vi "FPGA set up.vi"(6 "mirror cycles per frame":i16=256, 7 "enable external trigger":bool, 8 "lasersync":bool, 9 "bitfile name":T1, 10 "Start Delay (Ticks)":i16=1 min=1, 11 "resource name":T3) -> (0 "pixels per frame":i32, 3 "FPGA VI Reference Out":T2, 4 "Actual Depth 3":u32)   [LabVIEW 2012]
doc: "SciScan 1.2 160622"
uses:
  <vilib>/userdefined/High Color/nirio_resource_hc.ctl
  Custom Controls/FPGA reference typedef for 120MHz code.ctl
  Custom Controls/biotfile select.ctl
  <vilib>/FPGAPlugInAG/PXIe-7962R/niLvFpga_Open_PXIe-7962R.vi
  <vilib>/rvi/interface/common/dynamic/niFpgaDynamicAddResources.vi
  <vilib>/FPGAPlugInAG/PXIe-7961R/niLvFpga_Open_PXIe-7961R.vi
  <vilib>/FPGAPlugInAG/Dynamic/niLvFpga_Abort_Dynamic.vi
  <vilib>/Utility/error.llb/Error Cluster From Error Code.vi
  <vilib>/rvi/errors/niLvFpgaAdjustHostInterfaceError.vi
  <vilib>/FPGAPlugInAG/Dynamic/niLvFpga_Run_Dynamic.vi
  <vilib>/rvi/interface/nirviOpenFPGA/nirviOpenFPGA.xnode
  fpga bitfiles/7962with5751_512px_40Mhz.lvbitx
  fpga bitfiles/7962with5751_12kHz_512px_50MHz_4ch.lvbitx
  fpga bitfiles/7962with5751_512px_50Mhz.lvbitx
  fpga bitfiles/7961with5734_1024px_120Mhz or ext lasersync.lvbitx
  fpga bitfiles/7962with5734_1024px_120Mhz or ext lasersync.lvbitx
  fpga bitfiles/7962with5751_12kHz_1024px_2ch_50MHz.lvbitx
  fpga bitfiles/7962with5734_512px_120Mhz or ext lasersync.lvbitx
  fpga bitfiles/7961with5734_512px_120Mhz or ext lasersync.lvbitx
  fpga bitfiles/7962with5751_1536px_2ch_40Mhz.lvbitx
  fpga bitfiles/7962with5751_1536px_2ch_50Mhz.lvbitx
  <vilib>/rvi/interface/nirviMethod/nirviMethod.xnode
  <vilib>/rvi/interface/nirviReadWriteControl/nirviReadWriteControl.xnode
  <vilib>/rvi/errors/niLvFpgaMergeErrorWithErrorCode.vi
  <vilib>/FPGAPlugInAG/Dynamic/niLvFpga_ConfigureFifo_Dynamic.vi
  NiFpgaLv.dll
  <vilib>/rvi/interface/Simulation/niFpgaSimulationCallBeginRW.vi
panel:
  out "IO Module\\User Command Status":u8
  out "Array":bool[](array[boolean])
  in  "Requested Depth":u32=100000000
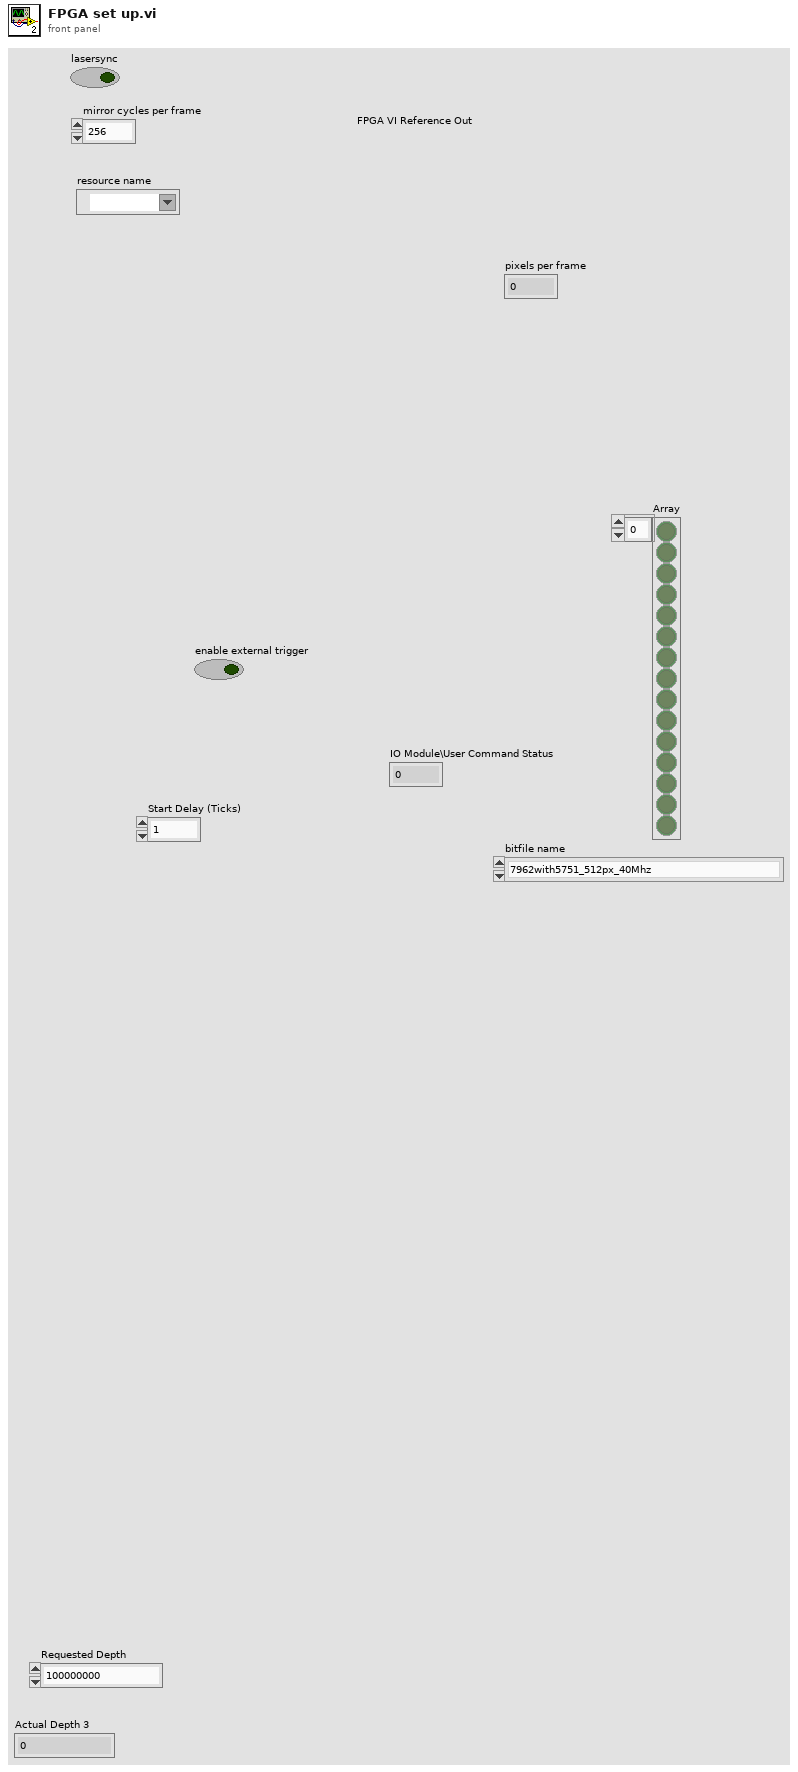
[diagram p1: front panel]
types:
  T1 = typedef "biotfile select.ctl" = enum16{"7962with5751_512px_40Mhz", "7962with5751_512px_50Mhz", "7961with5734_1024px_120Mhz or ext lasersync", "7962with5734_1024px_120Mhz or ext lasersync", "7962with5734_512px_120Mhz or ext lasersync", "7961with5734_512px_120Mhz or ext lasersync", "7962with5751_12kHz_512px_50MHz_4ch", "7962with5751_1536px_2ch_40Mhz", "7962with5751_1536px_2ch_50Mhz", "7962with5751_12kHz_1024px_2ch_50MHz"}
  T2 = typedef "FPGA reference typedef for 120MHz code.ctl" = refnum<k20>
  T3 = typedef "nirio_resource_hc.ctl" = tag
  T4 = cluster{"IO Module\\User Command":u8, "IO Module\\User Data 0":u8, "IO Module\\User Data 1":u8}
  T5 = cluster{"IO Module\\User Command":u8, "IO Module\\User Data 0":u8, "IO Module\\User Data 1":u8}[]
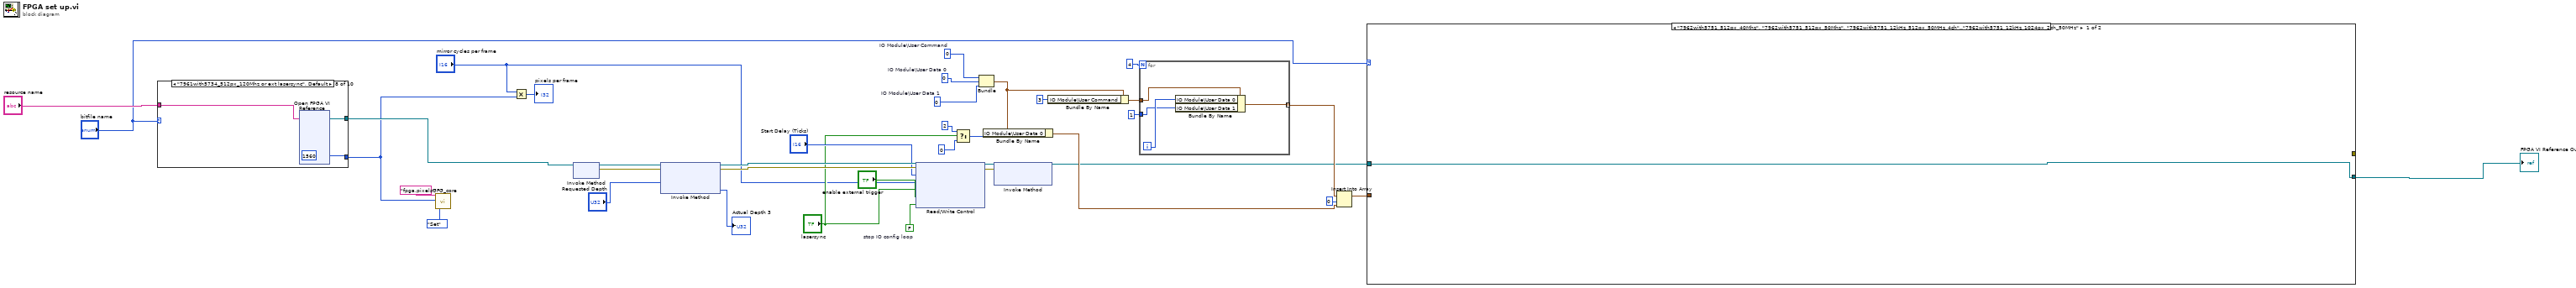
[diagram p0: block diagram]
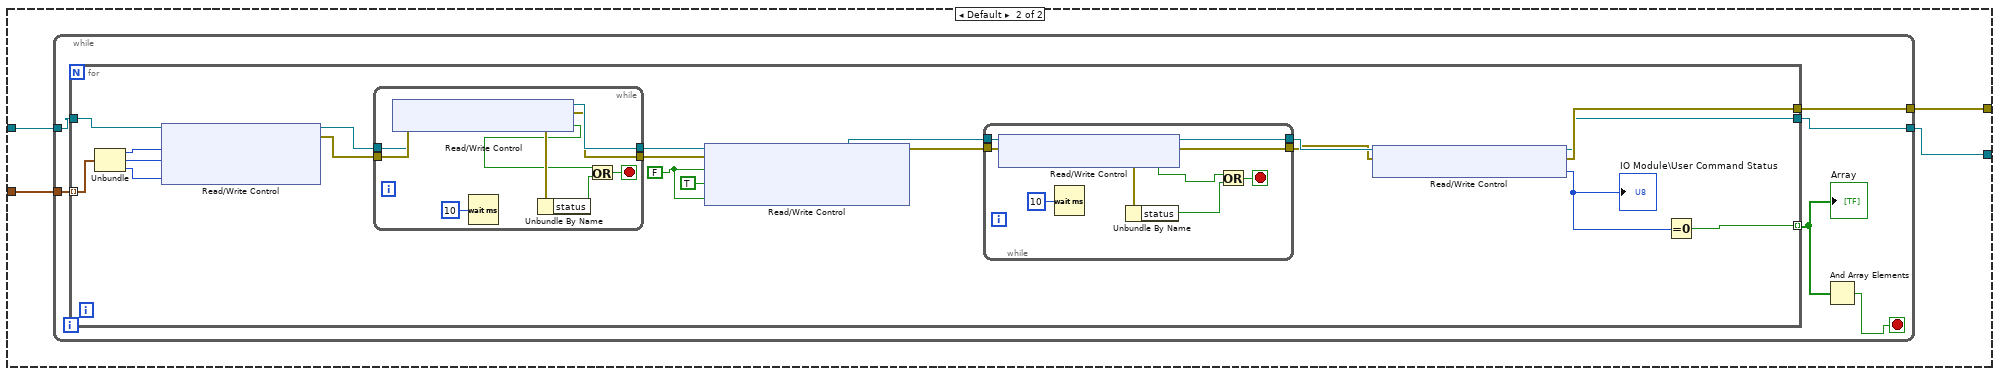
[diagram p2: hidden frame]
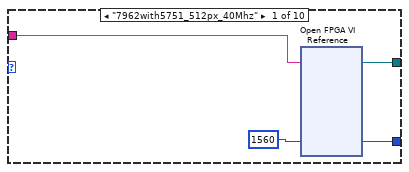
[diagram p3: hidden frame]
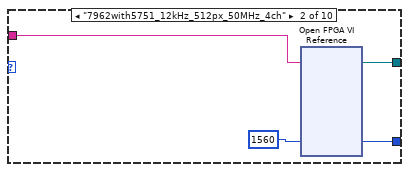
[diagram p4: hidden frame]
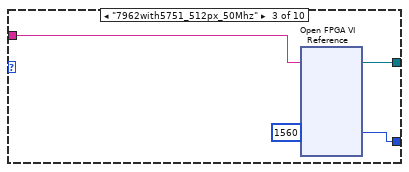
[diagram p5: hidden frame]
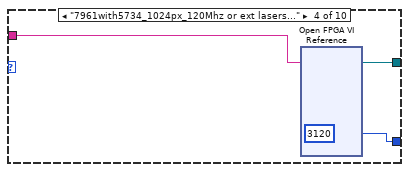
[diagram p6: hidden frame]
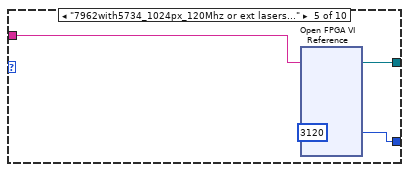
[diagram p7: hidden frame]
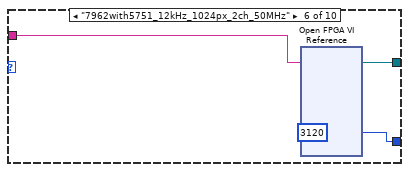
[diagram p8: hidden frame]
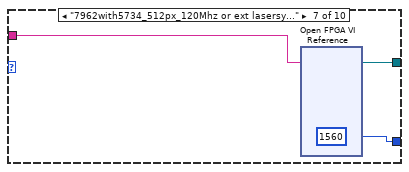
[diagram p9: hidden frame]
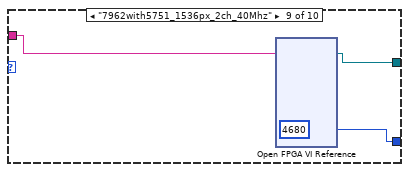
[diagram p10: hidden frame]
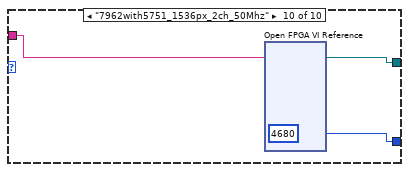
[diagram p11: hidden frame]
diagram:
  w24 = u8 0  # IO Module\User Data 1
  w25 = u8 0  # IO Module\User Data 0
  w26 = u8 0  # IO Module\User Command
  w27 = FALSE  # stop IO config loop
  n1 = case shown="\"7961with5734_512px_120Mhz or ext lasersync\", Default" "bitfile name" {
    tunnel: [w40 w43 w46 w49 w52 w55 w58 w61 w64 w67] -> w8
    tunnel: "resource name" -> [w39 w42 w45 w48 w51 w54 w57 w60 w62 w65]
    tunnel: [1560 1560 1560 3120 3120 3120 1560 1560 4680 4680] -> w3
    frame "7962with5751_512px_40Mhz" {
      n2 = xnode "Open FPGA VI Reference"("resource name"=w39) -> ("FPGA VI Reference Out"=w40:refnum<k20>)  [unwired: 1 in, 1 out]
    }
    frame "7962with5751_12kHz_512px_50MHz_4ch" {
      n3 = xnode "Open FPGA VI Reference"("resource name"=w42) -> ("FPGA VI Reference Out"=w43:refnum<k20>)  [unwired: 1 in, 1 out]
    }
    frame "7962with5751_512px_50Mhz" {
      n4 = xnode "Open FPGA VI Reference"("resource name"=w45) -> ("FPGA VI Reference Out"=w46:refnum<k20>)  [unwired: 1 in, 1 out]
    }
    frame "7961with5734_1024px_120Mhz or ext lasersync" {
      n5 = xnode "Open FPGA VI Reference"("resource name"=w48) -> ("FPGA VI Reference Out"=w49:refnum<k20>)  [unwired: 1 in, 1 out]
    }
    frame "7962with5734_1024px_120Mhz or ext lasersync" {
      n6 = xnode "Open FPGA VI Reference"("resource name"=w51) -> ("FPGA VI Reference Out"=w52:refnum<k20>)  [unwired: 1 in, 1 out]
    }
    frame "7962with5751_12kHz_1024px_2ch_50MHz" {
      n7 = xnode "Open FPGA VI Reference"("resource name"=w54) -> ("FPGA VI Reference Out"=w55:refnum<k20>)  [unwired: 1 in, 1 out]
    }
    frame "7962with5734_512px_120Mhz or ext lasersync" {
      n8 = xnode "Open FPGA VI Reference"("resource name"=w57) -> ("FPGA VI Reference Out"=w58:refnum<k20>)  [unwired: 1 in, 1 out]
    }
    frame "7961with5734_512px_120Mhz or ext lasersync", Default {
      n9 = xnode "Open FPGA VI Reference"("resource name"=w60) -> ("FPGA VI Reference Out"=w61:refnum<k20>)  [unwired: 1 in, 1 out]
    }
    frame "7962with5751_1536px_2ch_40Mhz" {
      n10 = xnode "Open FPGA VI Reference"("resource name"=w62) -> ("FPGA VI Reference Out"=w64:refnum<k20>)  [unwired: 1 in, 1 out]
    }
    frame "7962with5751_1536px_2ch_50Mhz" {
      n11 = xnode "Open FPGA VI Reference"("resource name"=w65) -> ("FPGA VI Reference Out"=w67:refnum<k20>)  [unwired: 1 in, 1 out]
    }
  }
  n12 = call "GFG_core.vi"("Variable Name in"="fpga.pixels", "Variant in"=w3, "Action"=enum16{"Init", "Set", "Get"}."Set") -> ()  [unwired: 10 in, 7 out]
  n13 = Multiply(x="mirror cycles per frame", y=w3) -> (x*y=→"pixels per frame":i32)
  n14 = xnode "Invoke Method"("FPGA VI Reference In"=w8) -> ("FPGA VI Reference Out"=w37:refnum<k20>, "error out"=w36:errorcluster)  [unwired: 1 in]
  n15 = xnode "Invoke Method"("FPGA VI Reference In"=w37, "error in"=w36, "Requested Depth"="Requested Depth") -> ("FPGA VI Reference Out"=w35:refnum<k20>, "error out"=w33:errorcluster, "Actual Depth"=→"Actual Depth 3":u32)
  n16 = xnode "Read/Write Control"("FPGA VI Reference In"=w35, "error in"=w33, "Start Delay (Ticks)"="Start Delay (Ticks)", "mirror cycles per frame"="mirror cycles per frame", "lasersync"="lasersync", "enable external trigger"="enable external trigger", "stop IO config loop"=w27) -> ("FPGA VI Reference Out"=w30:refnum<k20>, "error out"=w29:errorcluster)
  n17 = Select(t=u8 2 ("IO Module\\User Data 0"), s="lasersync", f=u8 0 ("IO Module\\User Data 0")) -> (s? t:f=w20:u8)
  n18 = Bundle("IO Module\\User Command"=w26, "IO Module\\User Data 0"=w25, "IO Module\\User Data 1"=w24) -> (w19:T4)  [unwired: 1 in]
  n19 = Bundle By Name(cluster=w19, "IO Module\\User Data 0"=w20) -> (w15:T4)
  n20 = xnode "Invoke Method"("FPGA VI Reference In"=w30, "error in"=w29) -> ("FPGA VI Reference Out"=w13:refnum<k20>)  [unwired: 1 in, 1 out]
  n21 = Bundle By Name(cluster=w19, "IO Module\\User Command"=u8 3 ("IO Module\\User Command")) -> (w17:T4)
  n22 = for {
    N: 4 -> [_]
    tunnel: w17 -> [w71]
    tunnel: 1 -> [w68]
    tunnel: [w70] -> w16 mode=indexing
    i -> [w69]
    n23 = Bundle By Name(cluster=w71, "IO Module\\User Data 0"=w69, "IO Module\\User Data 1"=w68) -> (w70:T4)
  }
  n24 = Insert Into Array(array=w16, index=0, new element=w15) -> (w12:T5)
  n25 = case shown="\"7962with5751_512px_40Mhz\", \"7962with5751_512px_50Mhz\", \"7962with5751_12kHz_512px_50MHz_4ch\"..\"7962with5751_12kHz_1024px_2ch_50MHz\"" "bitfile name" {
    tunnel: [_ w76] -> _
    tunnel: w13 -> [w72 w75]
    tunnel: w12 -> [_ w74]
    tunnel: [w72 w73] -> w2
    frame "7962with5751_512px_40Mhz", "7962with5751_512px_50Mhz", "7962with5751_12kHz_512px_50MHz_4ch".."7962with5751_12kHz_1024px_2ch_50MHz" {
    }
    frame Default {
      n26 = while {
        tunnel: w74 -> [w82]
        tunnel: [w80] -> w76
        tunnel: w75 -> [w79]
        tunnel: [w78] -> w73
        stop <- w77 stop-if-true
        n27 = for {
          tunnel: w82 -> [w96] mode=indexing
          tunnel: [w91] -> w81 mode=indexing
          tunnel: [w90] -> w80
          tunnel: w79 -> [w97]
          tunnel: [w85] -> w78
          w84 = FALSE ("Sample Clock Commit")
          n28 = Unbundle(w96) -> ("IO Module\\User Command"=w95:u8, "IO Module\\User Data 0"=w94:u8, "IO Module\\User Data 1"=w93:u8)
          n29 = xnode "Read/Write Control"("FPGA VI Reference In"=w97, "IO Module\\User Command"=w95, "IO Module\\User Data 0"=w94, "IO Module\\User Data 1"=w93) -> ("FPGA VI Reference Out"=w98:refnum<k20>, "error out"=w99:errorcluster)  [unwired: 1 in]
          n30 = while {
            tunnel: w98 -> [w113]
            tunnel: w99 -> [w114]
            tunnel: [w111] -> w87
            tunnel: [w112] -> w86
            stop <- w115 stop-if-true
            n31 = xnode "Read/Write Control"("FPGA VI Reference In"=w113, "error in"=w114) -> ("FPGA VI Reference Out"=w112:refnum<k20>, "error out"=w111:errorcluster, "IO Module\\User Command Idle"=w110:bool)
            n32 = Wait (ms)(milliseconds to wait=u32 10) -> ()  [unwired: 1 out]
            n33 = Unbundle By Name(w111) -> ("status"=w116:bool)
            n34 = Or(x=w110, y=w116) -> (x .or. y?=w115:bool)
          }
          n35 = xnode "Read/Write Control"("FPGA VI Reference In"=w86, "error in"=w87, "IO Module\\User Command Commit"=w84, "IO Module\\User Command Commit"=TRUE ("Sample Clock Commit"), "IO Module\\User Command Commit"=w84) -> ("FPGA VI Reference Out"=w88:refnum<k20>, "error out"=w89:errorcluster)
          n36 = while {
            tunnel: w88 -> [w105]
            tunnel: w89 -> [w106]
            tunnel: [w103] -> w100
            tunnel: [w104] -> w101
            stop <- w107 stop-if-true
            n37 = xnode "Read/Write Control"("FPGA VI Reference In"=w105, "error in"=w106) -> ("FPGA VI Reference Out"=w104:refnum<k20>, "error out"=w103:errorcluster, "IO Module\\User Command Idle"=w102:bool)
            n38 = Wait (ms)(milliseconds to wait=u32 10) -> ()  [unwired: 1 out]
            n39 = Unbundle By Name(w103) -> ("status"=w108:bool)
            n40 = Or(x=w102, y=w108) -> (x .or. y?=w107:bool)
          }
          n41 = xnode "Read/Write Control"("FPGA VI Reference In"=w101, "error in"=w100) -> ("FPGA VI Reference Out"=w85:refnum<k20>, "error out"=w90:errorcluster, "IO Module\\User Command Status"=w92:u8)
          "IO Module\\User Command Status" <- w92
          n42 = Equal To 0?(x=w92) -> (x = 0?=w91:bool)
        }
        "Array" <- w81
        n43 = And Array Elements(Boolean array=w81) -> (logical AND=w77:bool)
      }
    }
  }
  "FPGA VI Reference Out" <- w2
